vi "Alarm History.vi"(10 "user event":refnum<user-event>) -> ()   [LabVIEW 2021, in "Dynamic Shared Variables.lvlib"]
doc: "Displays the alarm history of the specified process."
uses:
  Dynamic Shared Variables.lvlib
  Alarm Description Item.ctl
  <vilib>/Platform/TimedLoop/XDataNode/timing_clust.ctl
  <vilib>/Platform/TimedLoop/XDataNode/nitl_modes.ctl
  <vilib>/Platform/TimedLoop/XDataNode/wakeup.ctl
  Tag VIs/Tag FGV Operation Enum.ctl
  support/Message Queue/Enqueue Message (Single).vi
  <vilib>/Platform/TimedLoop/XDataNode/XDataNode.xnode
  <vilib>/lvdsc/NI_DSC.lvlib
  support/Message Queue/Message Queue.lvlib
  <vilib>/Platform/TimedLoop/XDataNode/XDNodeRunTimeDep.lvlib
panel:
  in  "OK Button":bool
  in  "Sort":T1(ring)
  in  "Alarm Display Format":T2[](array[typedef])=[enum."alarm URL", enum."set time", enum."ack time", enum."alarm area", enum."priority"]
  in  "Alarm Summary":i32(listbox)=1
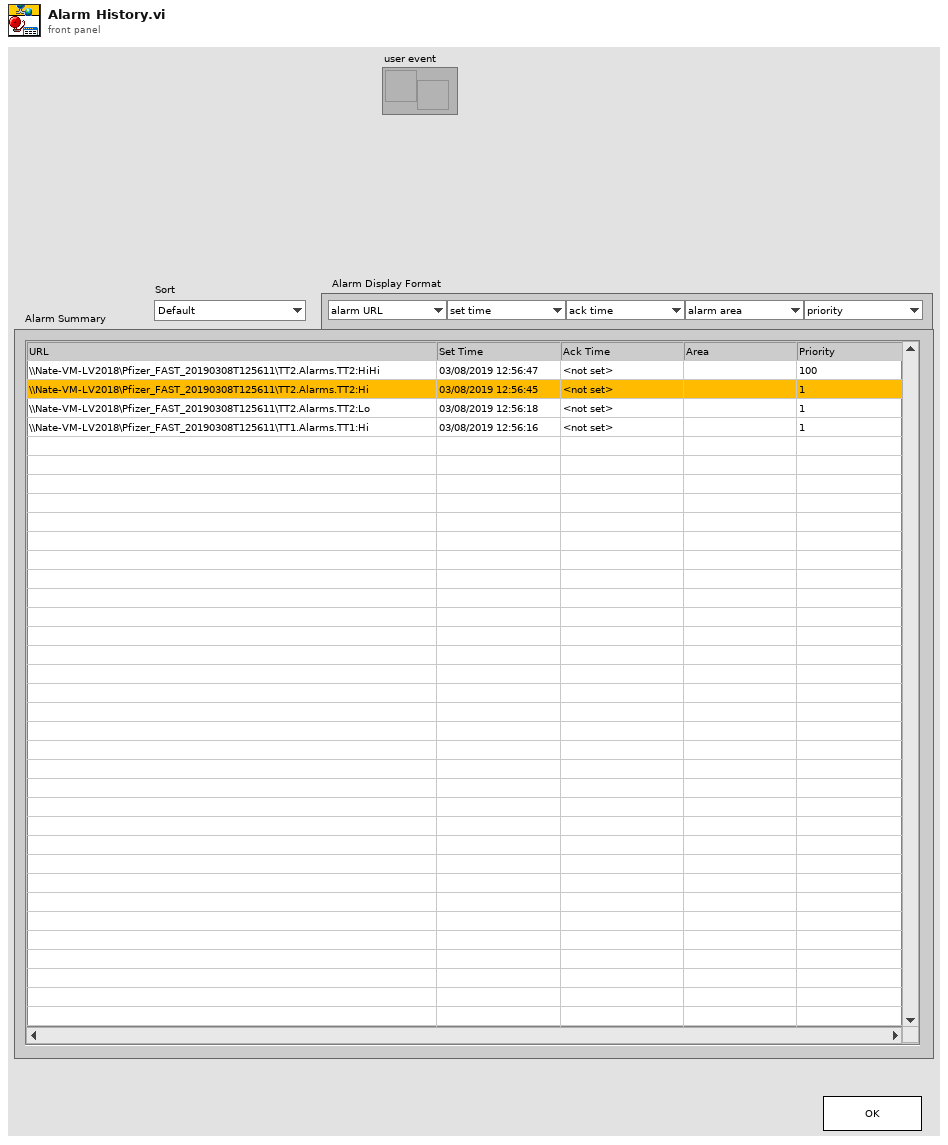
[diagram p1: front panel]
types:
  T1 = enum16{"Default", "Chronological", "Reverse Chronological"}
  T2 = typedef "Dynamic Shared Variables.lvlib/Alarm Description Item.ctl" = enum16{"alarm URL", "event?", "set time", "ack time", "clear time", "set user", "ack user", "clear user", "set point", "value", "priority", "alarm area", "alarm description", "ack comment"}
  T3 = cluster{"alarm URL":string, "set time":timestamp, "set user":string, "ack time":timestamp, "ack user":string, "clear time":timestamp, "clear user":string, "setpoint":dbl, "value":dbl, "priority":u32, "alarm area":string, "alarm description":string, "ack comment":string, "event?":bool, "Refnum":u64}[]
  T4 = typedef "XDNodeRunTimeDep.lvlib/timing_clust.ctl" = cluster{"Expected End [f-1]":u64, "Actual End [f-1]":u64, "Finished Late? [f-1]":bool, "Expected End [i-1]":u64, "Actual End [i-1]":u64, "Finished Late? [i-1]":bool, "Expected Start [i]":u64, "Actual Start [i]":u64, "Expected Start [f]":u64, "Actual Start [f]":u64, "Source Name":string, "Structure Name":string, "Period":i64, "Deadline":i64, "Offset":i64, "Start":i64, "Priority":i32, "Timeout":i32, "Mode":T5, "Wakeup Reason":T6, "Error":errorcluster, "Source Type":string, "Secondary Source Type":string, "Global End Time":u64, "Global Start Time":u64, "Frame Duration":u64, "Iteration Duration":u64, "Assigned CPU":i32, "I/O Scan Engine Mode":u32}
  T5 = typedef "XDNodeRunTimeDep.lvlib/nitl_modes.ctl" = enum32{"No Change", "Process missed periods, maintain original phase", "Discard missed periods, maintain original phase", "Process missed periods, ignore original phase", "Discard missed periods, ignore original phase"}
  T6 = typedef "XDNodeRunTimeDep.lvlib/wakeup.ctl" = enum32{"Normal", "Aborted", "Asynchronous wakeup", "Timing source error", "Timed loop error", "Timeout"}
  T7 = typedef "Tag FGV Operation Enum.ctl" = enum16{"Init", "Set Notification Queue", "Create Tag", "Commit", "Write Tag (Numeric)", "Write Tag (Boolean)", "Read All Tags", "Read One Tag", "Delete Tag Category", "Set Alarm Parameters (Numeric)", "Set Alarm Parameters (Boolean)", "Enable All Alarms", "Disable All Alarms", "Delete All Tags", "Read Alarms", "Ack Alarm", "Read Alarm Parameters (Numeric)", "Read Alarm Parameters (Boolean)"}
  T8 = cluster{"start timestamp":timestamp, "stop timestamp (now)":timestamp, "shared variable name":string, "process":string, "set user":string, "clear user":string, "ack user":string, "alarm area":string, "ack comment":string, "alarm description":string, "alarm setpoint":dbl, "value at alarm":dbl, "minimum priority":i32, "maximum priority":i32, "filter on...":cluster{"start timestamp":bool, "shared variable name":bool, "process":bool, "set user":bool, "clear user":bool, "ack user":bool, "alarm area":bool, "ack comment":bool, "alarm description":bool, "alarm setpoint":bool, "value at alarm":bool, "minimum priority":bool, "maximum results":bool, "return newest entries first":bool}, "show...":u16, "maximum results":i32, "return newest entries first":bool}
  T9 = cluster{"alarm URL":string, "set time":timestamp, "set user":string, "ack time":timestamp, "ack user":string, "clear time":timestamp, "clear user":string, "setpoint":dbl, "value":dbl, "priority":u32, "alarm area":string, "alarm description":string, "ack comment":string, "Refnum":u32, "event?":bool}[]
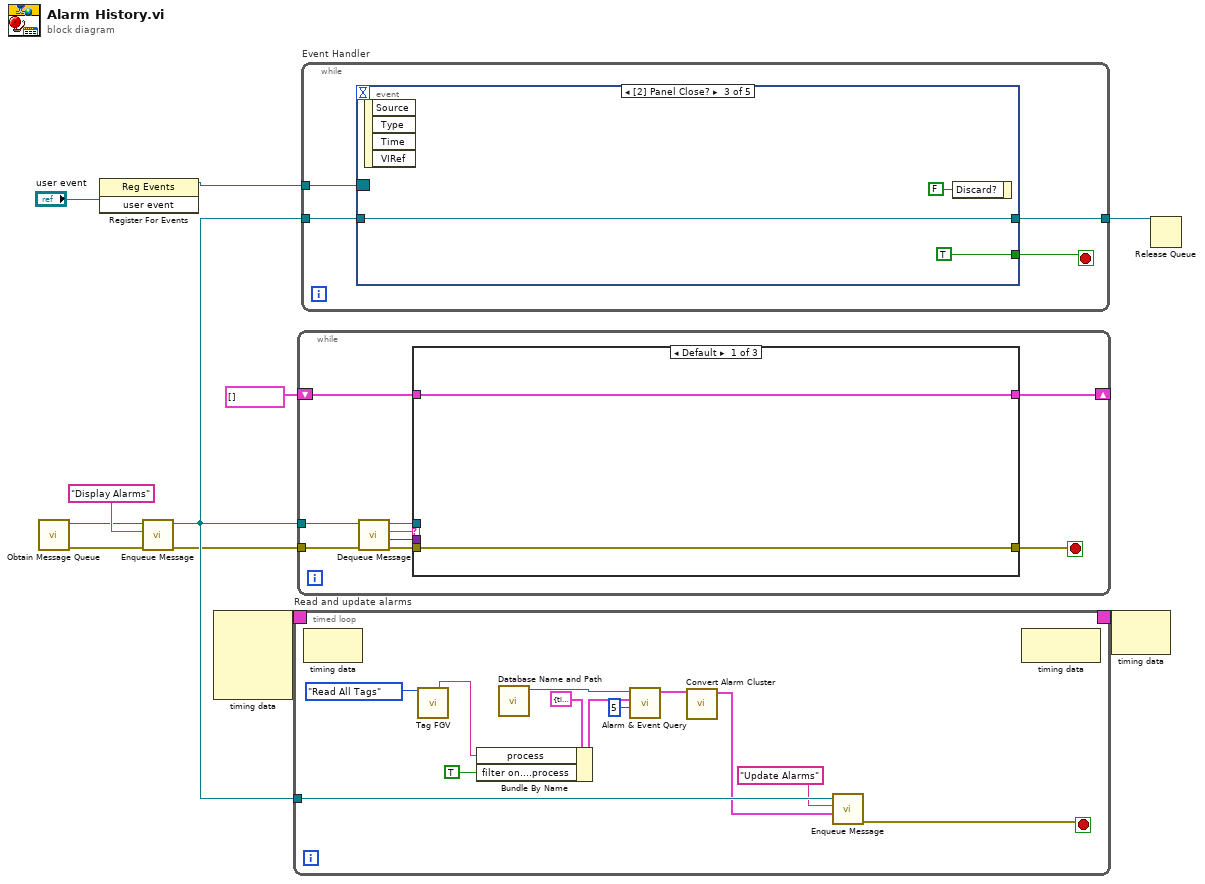
[diagram p0: block diagram]
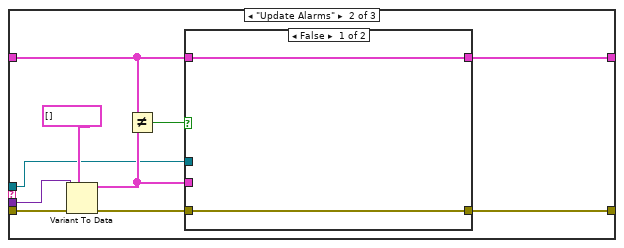
[diagram p2: hidden frame]
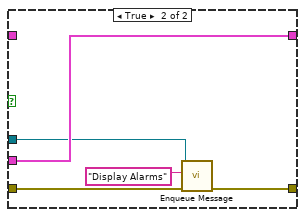
[diagram p3: hidden frame]
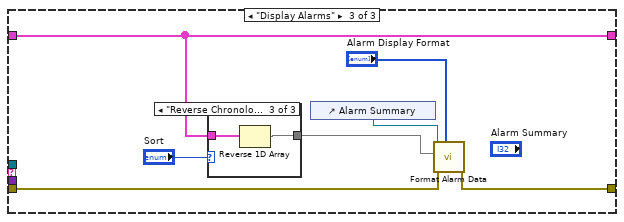
[diagram p4: hidden frame]
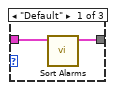
[diagram p5: hidden frame]
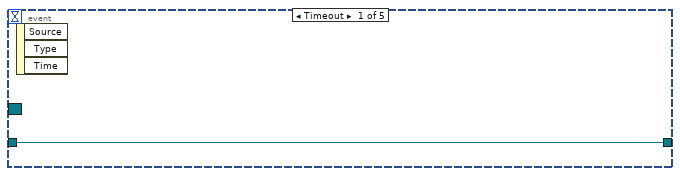
[diagram p7: hidden frame]
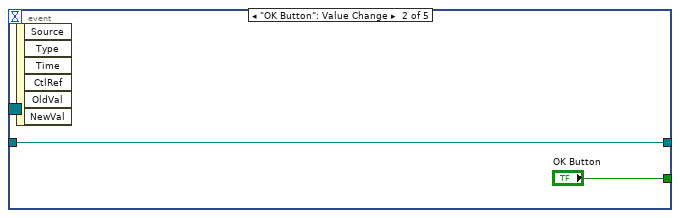
[diagram p8: hidden frame]
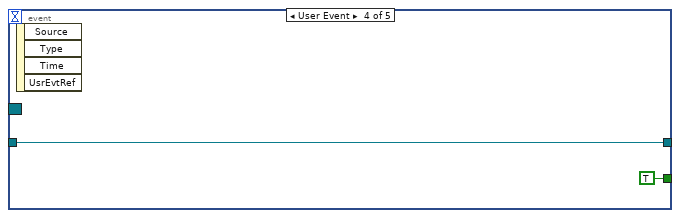
[diagram p9: hidden frame]
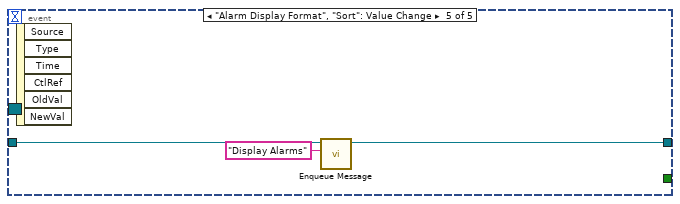
[diagram p10: hidden frame]
diagram:
  n1 = call "Obtain Message Queue.vi"() -> ("error out"=w4:errorcluster, "Message Queue"=w6:refnum<queue>)  [unwired: 10 in]
  n2 = register-events("user event") -> (reference out=w2:refnum<event-registration>)  [unwired: 2 in, 1 out]
  n3 = call-poly "Enqueue Message.vi"("error in (no error)"=w4, "Message"="Display Alarms", "Message Queue"=w6) -> ("error out"=w3:errorcluster, "dup Message Queue"=w5:refnum<queue>)  [unwired: 7 in]
  n4 = node-c288() -> (w11:T4)  [unwired: 4 in]
  n5 = timed-loop "Read and update alarms" {
    timing: w11 -> [_]
    timing-out: [_] -> w10
    tunnel: w5 -> [w17]
    stop <- w14 stop-if-true
    n6 = node-c288() -> ()  [unwired: 1 in, 1 out]
    n7 = call "Tag FGV.vi"("Operation"=Tag_FGV_Operation_Enum."Read All Tags") -> ("Process Name"=w12:string)  [unwired: 7 in, 7 out]
    n8 = Bundle By Name(cluster=T8 {"start timestamp"=timestamp(0 s since 1904-01-01), "stop timestamp (now)"=timestamp(0 s since 1904-01-01), "shared variable name"="", "process"="", "set user"="", "clear user"="", "ack user"="", "alarm area"="", "ack comment"="", "alarm description"="", "alarm setpoint"=0.0, "value at alarm"=0.0, "minimum priority"=-1, "maximum priority"=-1, "filter on..."={"start timestamp"=FALSE, "shared variable name"=FALSE, "process"=FALSE, "set user"=FALSE, "clear user"=FALSE, "ack user"=FALSE, "alarm area"=FALSE, "ack comment"=FALSE, "alarm description"=FALSE, "alarm setpoint"=FALSE, "value at alarm"=FALSE, "minimum priority"=FALSE, "maximum results"=FALSE, "return newest entries first"=FALSE}, "show..."=0, "maximum results"=-1, "return newest entries first"=FALSE} ("filter"), "process"=w12, "filter on....process"=TRUE) -> (w22:T8)
    n9 = call "Database Name and Path.vi"() -> ("databse path"=w20:path)  [unwired: 9 in, 2 out]
    n10 = call <vilib>:"Alarm & Event Query.vi"("timeout (30 s)"=5, "filter"=w22, "database URL"=w20) -> ("alarm data"=w19:T9)  [unwired: 6 in, 2 out]
    n11 = call "Convert Alarm Cluster.vi"("alarm data in"=w19) -> ("alarms out"=w15:T3)  [unwired: 10 in]
    n12 = call-poly "Enqueue Message.vi"("Message Data"=w15, "Message"="Update Alarms", "Message Queue"=w17) -> ("error out"=w14:errorcluster)  [unwired: 7 in, 1 out]
    n13 = node-c288() -> ()  [unwired: 1 in, 1 out]
  }
  n14 = while {
    tunnel: w5 -> [w33]
    tunnel: w3 -> [w32]
    shift-right: [w29] -> _
    shift-left: T3 [] ("alarms out") -> [w31]
    stop <- w26 stop-if-true
    n15 = call "Dequeue Message.vi"("error in (no error)"=w32, "Message Queue"=w33) -> ("error out"=w28:errorcluster, "Message Data"=w30:variant, "Message"=w34:string, "dup Message Queue"=w27:refnum<queue>)  [unwired: 6 in]
    n16 = case shown="Default" w34 {
      tunnel: w31 -> [w36 w41 w59]
      tunnel: w30 -> [_ w45 _]
      tunnel: [w36 w43 w59] -> w29
      tunnel: w28 -> [w35 w40 w55]
      tunnel: [w35 w38 w54] -> w26
      tunnel: w27 -> [_ w37 _]
      frame Default {
      }
      frame "Update Alarms" {
        n17 = Variant To Data(error in=w40, type=T3 [] ("alarms out"), Variant=w45) -> (data=w42:T3, error out=w39:errorcluster)
        n18 = Not Equal?(x=w41, y=w42) -> (x != y?=w44:bool)
        n19 = case shown="False" w44 {
          tunnel: [w47 w50] -> w43
          tunnel: w42 -> [_ w50]
          tunnel: w41 -> [w47 _]
          tunnel: w39 -> [w48 w52]
          tunnel: [w48 w51] -> w38
          tunnel: w37 -> [_ w49]
          frame False {
          }
          frame True {
            n20 = call-poly "Enqueue Message.vi"("error in (no error)"=w52, "Message"="Display Alarms", "Message Queue"=w49) -> ("error out"=w51:errorcluster)  [unwired: 7 in, 1 out]
          }
        }
      }
      frame "Display Alarms" {
        n21 = case shown="\"Reverse Chronological\"" "Sort" {
          tunnel: w59 -> [w62 w63 w65]
          tunnel: [w61 w63 w64] -> w56
          frame "Default" {
            n22 = call "Sort Alarms.vi"("alarms"=w62) -> ("alarms out"=w61:T3)  [unwired: 10 in]
          }
          frame "Chronological" {
          }
          frame "Reverse Chronological" {
            n23 = Reverse 1D Array(array=w65) -> (reversed array=w64:T3)
          }
        }
        n24 = control-ref of="Alarm Summary"() -> (w57:refnum<vi>)
        n25 = call "Format Alarm Data.vi"("Alarm Display Format"="Alarm Display Format", "Error In"=w55, "alarm instances"=w56, "Multicolumn Listbox"=w57) -> ("Error Out"=w54:errorcluster)  [unwired: 4 in, 3 out]
      }
    }
  }
  n26 = while "Event Handler" {
    tunnel: w5 -> [w68]
    tunnel: [w67] -> w8
    tunnel: w2 -> [w66]
    stop <- w69 stop-if-true
    n27 = event shown="[2] Panel Close?" {
      selector: w66 -> [_ _ _ _ _]
      dyn-events: _ -> [_ _ _ _ _]
      timeout: _ -> [_ _ _ _ _]
      tunnel: [_ "OK Button" TRUE ("OK Button") TRUE ("OK Button") _] -> w69
      tunnel: w68 -> [w70 w71 w75 w77 w80]
      tunnel: [w70 w71 w75 w77 w78] -> w67
      event Timeout {
        n28 = event-data() -> ()  [unwired: 1 in, 3 out]
      }
      event "OK Button": Value Change {
        n29 = event-data() -> ()  [unwired: 1 in, 6 out]
      }
      event Panel Close? {
        n30 = event-data() -> ()  [unwired: 1 in, 4 out]
        n31 = event-data("Discard?"=FALSE) -> ()  [unwired: 1 in, 1 out]
      }
      event User Event {
        n32 = event-data() -> ()  [unwired: 1 in, 4 out]
      }
      event "Alarm Display Format", "Sort": Value Change {
        n33 = event-data() -> ()  [unwired: 1 in, 6 out]
        n34 = call-poly "Enqueue Message.vi"("Message"="Display Alarms", "Message Queue"=w80) -> ("dup Message Queue"=w78:refnum<queue>)  [unwired: 8 in, 1 out]
      }
    }
  }
  n35 = node-c288(w10) -> ()  [unwired: 1 out]
  n36 = Release Queue(queue=w8) -> ()  [unwired: 2 in, 3 out]
